vi "右侧填充字符串.vi"(2 "Pad Character (\\s)":string=" ", 7 "String In":string, 13 "End Length":i32) -> (8 "String Out":string)   [LabVIEW 2012]
doc: "This VI adds as many pad characters as necessary to <B>String In</B> to give it a length of <B>End Length</B>.\n\nFreeware from Moore Good Ideas, www.mooregoodideas.com. Do not remove this line."
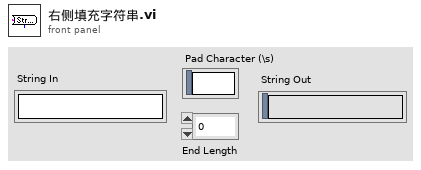
[diagram p1: front panel]
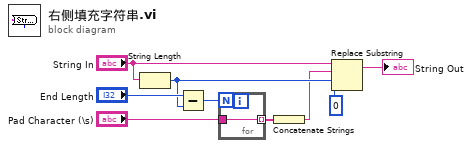
[diagram p0: block diagram]
diagram:
  n1 = String Length(string="String In") -> (length=w6:i32)
  n2 = Subtract(x="End Length", y=w6) -> (x-y=w4:i32)
  n3 = for {
    N: w4 -> [_]
    tunnel: "Pad Character (\\s)" -> [w10]
    tunnel: [w10] -> w2 mode=indexing
  }
  n4 = Concatenate Strings(w2) -> (w1:string)
  n5 = Replace Substring(2:0 ("length (len. of substring)"), 3:w6, 4:w1, 5:"String In") -> (1:→"String Out":string)  [unwired: 1 out]
